vi "Register Menu Events.vi"(8 "error in (no error)":errorcluster, 11 "Picture in":refnum<vi>) -> (0 "error out":errorcluster, 1 "CB VIs":refnum<vi>[](array[refnum]), 2 "event callback refnum":refnum<k27>, 3 "Cluster":T1)   [LabVIEW 2015, in "LV Image Editor Framework.lvlib" / "Image Editor Handler.lvclass"]
uses:
  Image Editor Handler.lvclass
  <vilib>/Utility/miscctls.llb/LVPoint32TypeDef.ctl
  Callbacks/Handler UI Callbacks.lvlib
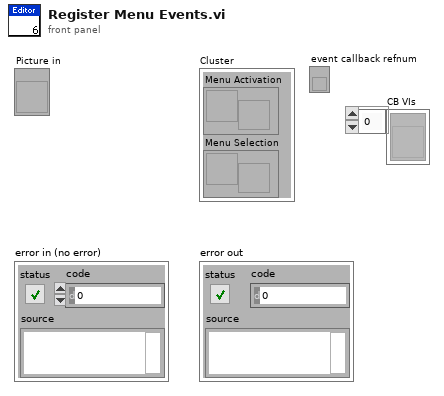
[diagram p1: front panel]
types:
  T1 = cluster{"Menu Activation":refnum<user-event>, "Menu Selection":refnum<user-event>}
  T2 = typedef "LVPoint32TypeDef.ctl" = cluster{"Horizontal":i32, "Vertical":i32}
  T3 = cluster{"ItemTag":string, "ItemPath":string, "Coords":T2, "SubObj":refnum<vi>}
  T4 = cluster{"Ack":refnum<k4>, "Shortcut Act. Data":cluster{"MenuRef":refnum<k9>, "Coords":T2, "SubObj":refnum<vi>}}
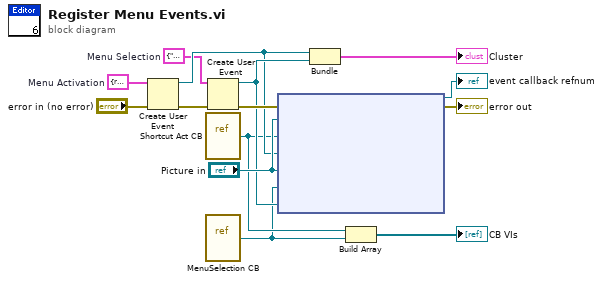
[diagram p0: block diagram]
diagram:
  w6 = T3 {"ItemTag"="", "ItemPath"="", "Coords"={"Horizontal"=0, "Vertical"=0}, "SubObj"=refnum}  # Menu Selection
  w5 = T4 {"Ack"=refnum, "Shortcut Act. Data"={"MenuRef"=refnum, "Coords"={"Horizontal"=0, "Vertical"=0}, "SubObj"=refnum}}  # Menu Activation
  n1 = Create User Event(user event datatype=w5, error in="error in (no error)") -> (user event=w7:refnum<user-event>, error out=w11:errorcluster)
  n2 = vi-ref "Shortcut Act CB.vi"() -> ("vi reference"=w3:refnum<vi>)
  n3 = vi-ref "MenuSelection CB.vi"() -> ("vi reference"=w2:refnum<vi>)
  n4 = Create User Event(user event datatype=w6, error in=w11) -> (user event=w8:refnum<user-event>, error out=w12:errorcluster)
  n5 = node(w12, "Picture in", w3, w7, "Picture in", w2, w8) -> (→"event callback refnum":refnum<k27>, →"error out":errorcluster)  [unwired: 1 in]
  n6 = Bundle("Menu Activation"=w7, "Menu Selection"=w8) -> (→"Cluster":T1)  [unwired: 1 in]
  n7 = Build Array(w3, w2) -> (→"CB VIs":refnum<vi>[])
